vi "Tx Construct.vi"(8 "error in":errorcluster, 10 "command words":T1[](array[typedef]), 11 "id":string) -> (0 "error out":errorcluster, 3 "Tx Execution Unit Implementation out":refnum<class "Tx Execution Unit.lvclass">)   [LabVIEW 2020, in "Ballard MIL-STD-1553 Engine.lvlib" / "Implementation.lvlib" / "Tx Execution Unit.lvclass"]
uses:
  Tx Execution Unit.lvclass
  Shared/Command Word.ctl
  C:/dev/niveristand-ballard-milStd1553-custom-device/Source/Custom Device Support/Engine/Implementation/Execution Unit/Execution Unit.lvclass
  Execution Unit/Execution Unit.lvclass/Execution Unit.ctl
  Execution Unit/Execution Unit.lvclass
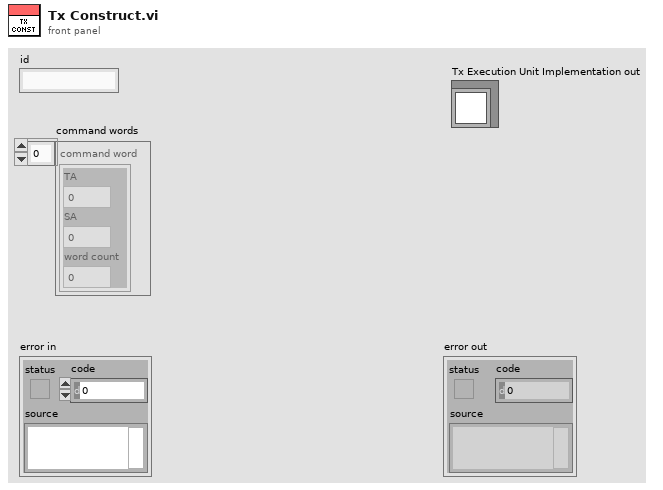
[diagram p1: front panel]
types:
  T1 = typedef "Command Word.ctl" = cluster{"TA":i8, "SA":i8, "word count":i8}
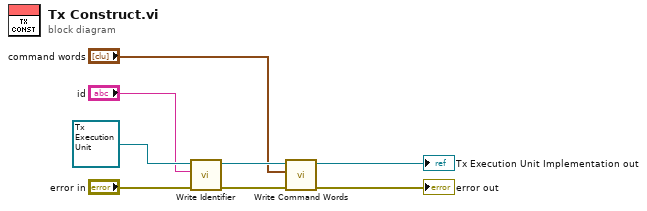
[diagram p0: block diagram]
diagram:
  n1 = call "Write Identifier.vi"("error in"="error in", "id"="id", "Execution Unit in"=refnum<class "Tx Execution Unit.lvclass"> refnum ("Communication Bus Template Interfaces:Implementation.lvlib:Tx Execution Unit.lvclass")) -> ("error out"=w8:errorcluster, "Execution Unit out"=w7:refnum<class "Tx Execution Unit.lvclass">)  [unwired: 7 in]
  n2 = call "Write Command Words.vi"("error in"=w8, "command words"="command words", "Execution Unit in"=w7) -> ("error out"=→"error out":errorcluster, "Execution Unit out"=→"Tx Execution Unit Implementation out":refnum<class "Tx Execution Unit.lvclass">)  [unwired: 7 in]
